vi "solar Create (Addons).vi"(8 "error in (no error)":errorcluster, 10 "AddonVIs":refnum<vi>[](array[refnum]), 11 "Default LVClass":refnum<class "solar.lvclass">) -> (0 "error out":errorcluster, 3 "solar out":refnum<class "solar.lvclass">)   [LabVIEW 2018, in "solar.lvclass"]
doc: "This initializes the SOLAR addons and launches the addons with '[startup]' or '[startup-only]' in the addon VI descriptions. SOLAR addons are loaded in the Tools menu."
uses:
  solar.lvclass
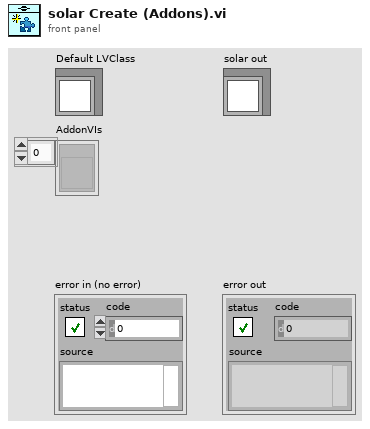
[diagram p1: front panel]
types:
  T1 = typedef "solar_ctl SOLAR Refnum.ctl" = refnum<k1>
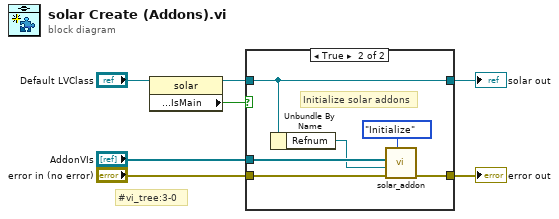
[diagram p0: block diagram]
diagram:
  # "#vi_tree:3-0"
  n1 = property class="solar"(reference="Default LVClass") -> (reference out=w4:refnum<class "solar.lvclass">, "Accessors:Main.IsMain"=w2:bool)  [unwired: 1 in, 1 out]
  n2 = case shown="True" w2 {
    tunnel: "error in (no error)" -> [w8 w14]
    tunnel: "AddonVIs" -> [_ w13]
    tunnel: w4 -> [w9 w10]
    tunnel: [w8 w11] -> w3
    tunnel: [w9 w10] -> w1
    frame False {
    }
    frame True {
      # "Initialize solar addons"
      n3 = Unbundle By Name(w10) -> ("Refnum"=w12:T1)
      n4 = call "solar_addon.vi"("Action (Launch)"=enum8{"Launch", "Initialize", "Shutdown"}."Initialize", "error in (no error)"=w14, "SOLAR Refnum"=w12, "AddonVIs (Initialize only)"=w13) -> ("error out"=w11:errorcluster)  [unwired: 6 in, 1 out]
    }
  }
  "error out" <- w3
  "solar out" <- w1
